vi "onKeyRead.vi"(7 "Qualified Name":string[](array[string]), 8 "error in (no error)":errorcluster, 10 "Keys":string[](array[string]), 11 "ConfigManager.Text.INI in":refnum<class "ConfigManager.Text.INI.lvclass">) -> (0 "error out":errorcluster, 2 "Keys out":string[](array[string]), 3 "ConfigManager.Text.INI out":refnum<class "ConfigManager.Text.INI.lvclass">, 5 "Qualified Name out":string[](array[string]))   [LabVIEW 2013, in "CfgManager.Text.lvlib" / "ConfigManager.Text.INI.lvclass"]
uses:
  ConfigManager.Text.INI.lvclass
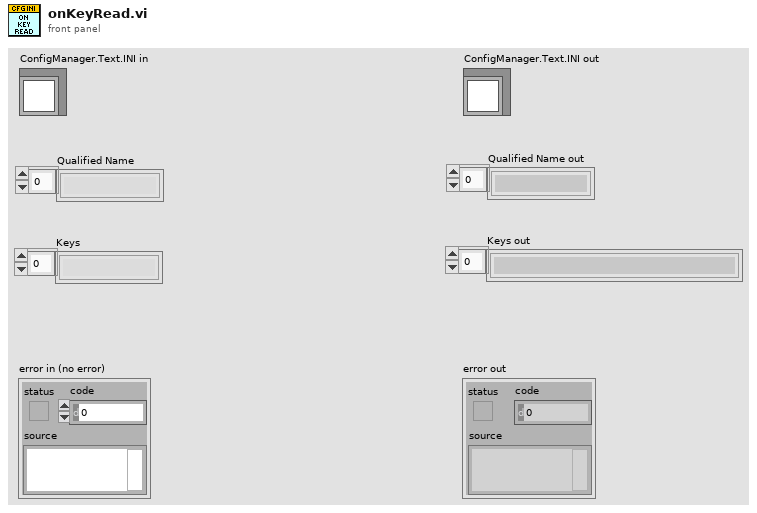
[diagram p1: front panel]
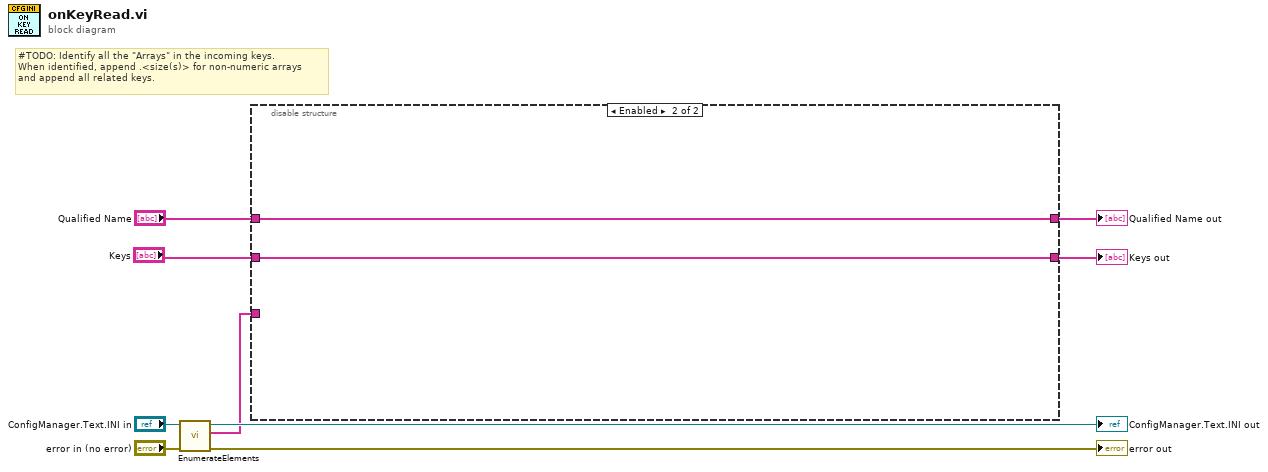
[diagram p0: block diagram]
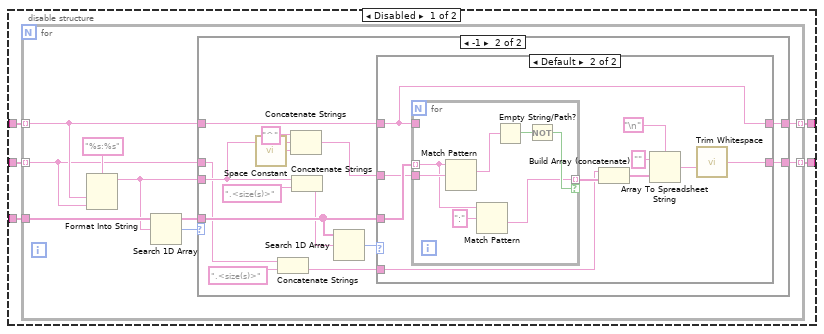
[diagram p2: hidden frame]
diagram:
  # "#TODO: Identify all the \"Arrays\" in the incoming keys.\nWhen identified, append .<size(s)> for non-numeric arrays\nand append all related keys."
  n1 = call-dynamic "EnumerateElements.vi"("error in (no error)"="error in (no error)", "ConfigManager.Text in"="ConfigManager.Text.INI in") -> ("error out"=→"error out":errorcluster, "keys"=w1:string[], "ConfigManager.Text out"=→"ConfigManager.Text.INI out":refnum<class "ConfigManager.Text.INI.lvclass">)  [unwired: 7 in]
  n2 = disable-structure shown="Enabled" {
    disable-tunnel: "Qualified Name" -> [w14 w57]
    disable-tunnel: [w13 w57] -> w4
    disable-tunnel: [w12 w56] -> w3
    disable-tunnel: "Keys" -> [w11 w56]
    disable-tunnel: w1 -> [w10 _]
    frame Disabled {
      n3 = for {
        tunnel: w10 -> [w18]
        tunnel: w14 -> [w16] mode=indexing
        tunnel: [w20] -> w13 mode=indexing
        tunnel: w11 -> [w15] mode=indexing
        tunnel: [w19] -> w12 mode=indexing
        n4 = Format Into String(format string="%s:%s", w16, w15) -> (resulting string=w17:string)  [unwired: 2 in, 1 out]
        n5 = Search 1D Array(1D array=w18, element=w17) -> (index of element=w21:i32)  [unwired: 1 in]
        n6 = case shown="-1" w21 {
          tunnel: w16 -> [w24 w38]
          tunnel: [w24 w37] -> w20
          tunnel: w15 -> [w23 w27]
          tunnel: [w23 w36] -> w19
          tunnel: w18 -> [_ w34]
          tunnel: w17 -> [_ w32]
          frame Default {
          }
          frame -1 {
            n7 = call <vilib>:"Space Constant.vi"() -> ("String"=w25:string)
            n8 = Concatenate Strings(w27, ".<size(s)>" ("string")) -> (w26:string)
            n9 = Concatenate Strings("^" ("string"), w32, w25) -> (w30:string)
            n10 = Concatenate Strings(w32, ".<size(s)>" ("string")) -> (w29:string)
            n11 = Search 1D Array(1D array=w34, element=w29) -> (index of element=w33:i32)  [unwired: 1 in]
            n12 = case shown="Default" w33 {
              tunnel: w38 -> [_ w44]
              tunnel: [_ w44] -> w37
              tunnel: [_ w39] -> w36
              tunnel: w34 -> [_ w48]
              tunnel: w30 -> [_ w47]
              tunnel: w26 -> [_ w45]
              frame -1 {
              }
              frame Default {
                n13 = for {
                  tunnel: w47 -> [w53]
                  tunnel: w48 -> [w51] mode=indexing
                  tunnel: [w49] -> w46 mode=indexing if=w52
                  tunnel: w44 -> [_]
                  n14 = Match Pattern(string=w51, regular expression=w53) -> (match substring=w55:string)  [unwired: 1 in, 3 out]
                  n15 = Match Pattern(string=w51, regular expression=":") -> (after substring=w49:string)  [unwired: 1 in, 3 out]
                  n16 = Empty String/Path?(string/path=w55) -> (empty?=w54:bool)
                  n17 = Not(x=w54) -> (.not. x?=w52:bool)
                }
                n18 = Build Array (concatenate)(w45, w46) -> (w43:string[])
                n19 = Array To Spreadsheet String(delimiter (Tab)="\n", array=w43, 3:"" ("format string")) -> (spreadsheet string=w40:string)
                n20 = call <vilib>:"Trim Whitespace.vi"("string"=w40) -> ("trimmed string"=w39:string)  [unwired: 1 in]
              }
            }
          }
        }
      }
    }
    frame Enabled {
    }
  }
  "Keys out" <- w3
  "Qualified Name out" <- w4
